vi "Constructor.vi"(8 "error in":errorcluster, 9 "Value":u8, 10 "Name":string, 11 "UnsignedByte in":refnum<class "UnsignedByte.lvclass">) -> (0 "error out":errorcluster, 3 "UnsignedByte out":refnum<class "UnsignedByte.lvclass">)   [LabVIEW 2021, in "ProligentXMLGenerator.lvlib" / "UnsignedByte.lvclass"]
uses:
  UnsignedByte.lvclass
  UnsignedByte.lvclass/UnsignedByte.ctl
  Attribute/Attribute.lvclass
  C:/Projects/proligent-xml-generator-labview/src/ProligentXMLGenerator/Base/Attribute/Attribute.lvclass
  C:/Projects/proligent-xml-generator-labview/src/ProligentXMLGenerator/Base/UnsignedByte/UnsignedByte.lvclass
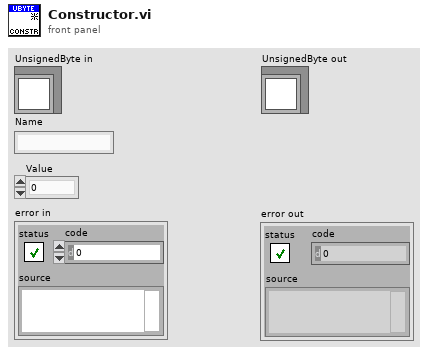
[diagram p1: front panel]
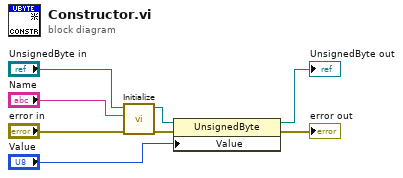
[diagram p0: block diagram]
diagram:
  n1 = call "Initialize.vi"("error in"="error in", "Name"="Name", "Attribute in"="UnsignedByte in") -> ("error out"=w4:errorcluster, "Attribute out"=w3:refnum<class "UnsignedByte.lvclass">)  [unwired: 7 in]
  n2 = property on="Property Node" class="UnsignedByte"(reference=w3, error in=w4, "Value"="Value") -> (reference out=→"UnsignedByte out":refnum<class "UnsignedByte.lvclass">, error out=→"error out":errorcluster)
